vi "Get Intensity Graph Cursor Position.vi"(9 "Ref In":refnum<vi>) -> (0 "Y Min":dbl format="%#_f", 1 "Y Max":dbl format="%#_f", 2 "X Min":dbl format="%#_f", 3 "X Max":dbl format="%#_f")   [LabVIEW 2024]
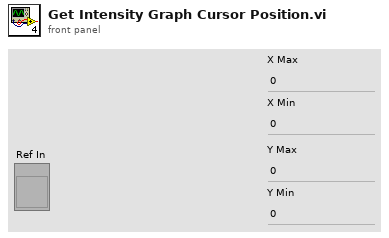
[diagram p1: front panel]
types:
  T1 = typedef "LVCursorListTypeDef.ctl" = cluster{"Name":string, "Color":u32, "Style":u8, "Point Style":u8, "Name Visible":bool, "Allow Drag":bool, "Cursor Mode":u32, "Plot":i32, "Index":i32, "Position":cluster{"X":dbl, "Y":dbl}, "X Scale":u32, "Y Scale":u32, "Watch Plots":i32[], "Watch All Plots":bool, "Plot Area":i32, "Label Offset":cluster{"X":dbl, "Y":dbl}}[]
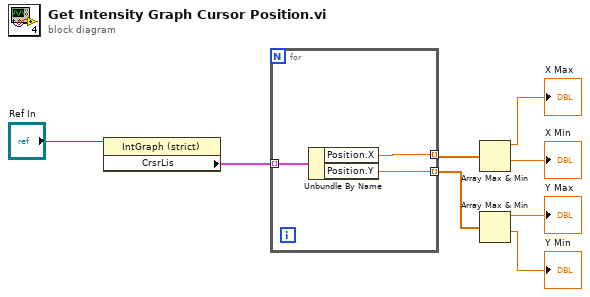
[diagram p0: block diagram]
diagram:
  n1 = property class="IntGraph (strict)"(reference="Ref In") -> ("CrsrLis"=w7:T1)  [unwired: 1 in, 2 out]
  n2 = for {
    tunnel: w7 -> [w11] mode=indexing
    tunnel: [w10] -> w6 mode=indexing
    tunnel: [w9] -> w5 mode=indexing
    n3 = Unbundle By Name(w11) -> ("Position.X"=w10:dbl, "Position.Y"=w9:dbl)
  }
  n4 = Array Max & Min(array=w6) -> (max value=→"X Max":dbl, min value=→"X Min":dbl)  [unwired: 2 out]
  n5 = Array Max & Min(array=w5) -> (max value=→"Y Max":dbl, min value=→"Y Min":dbl)  [unwired: 2 out]
